vi "Closedown.vi"(8 "error In":errorcluster, 10 "DeviceKey In":string, 11 "CmdLib In":refnum<k24>) -> (0 "error out":errorcluster)   [LabVIEW 2013]
uses:
  C:/GEECS/Developers Version/source/Device Driver/Picomotor8742dotNet/NewFocus/CmdLib.dll
  CmdLib.dll
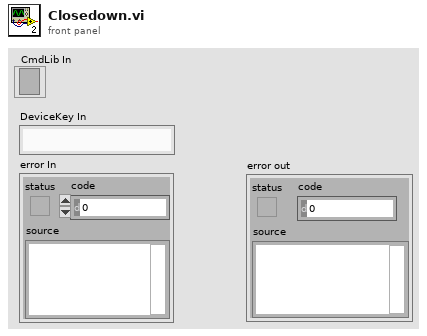
[diagram p1: front panel]
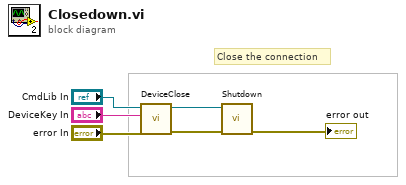
[diagram p0: block diagram]
diagram:
  # "Close the connection"
  n1 = call "DeviceClose.vi"("error in (no error)"="error In", "DeviceKey In"="DeviceKey In", "CmdLib In"="CmdLib In") -> ("error out"=w6:errorcluster, "CmdLib Out"=w4:refnum<k24>)  [unwired: 2 in, 1 out]
  n2 = call "Shutdown.vi"("error in (no error)"=w6, "CmdLib In"=w4) -> ("error out"=→"error out":errorcluster)  [unwired: 4 in, 1 out]
